vi "Multiple Files Handler.vi"(8 "Error In":errorcluster, 11 "TDMS Log":refnum<class "TDMS Logger.lvclass">) -> (0 "Error Out":errorcluster, 3 "TDMS Log Out":refnum<class "TDMS Logger.lvclass">)   [LabVIEW 2019, in "TDMS Logger.lvlib" / "TDMS Logger.lvclass"]
uses:
  TDMS Logger.lvclass
  TDMS Logger.lvclass/TDMS Logger.ctl
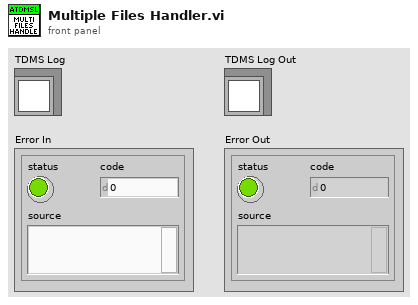
[diagram p1: front panel]
types:
  T1 = typedef "TDMS Logger.lvlib/TDMS Logger.lvclass/Multiple Files Action.ctl" = enum16{"Seperate based on size", "Seperate based on time", "Single file"}
  T2 = enum16{"open", "open or create", "create or replace", "create", "open (read-only)"}
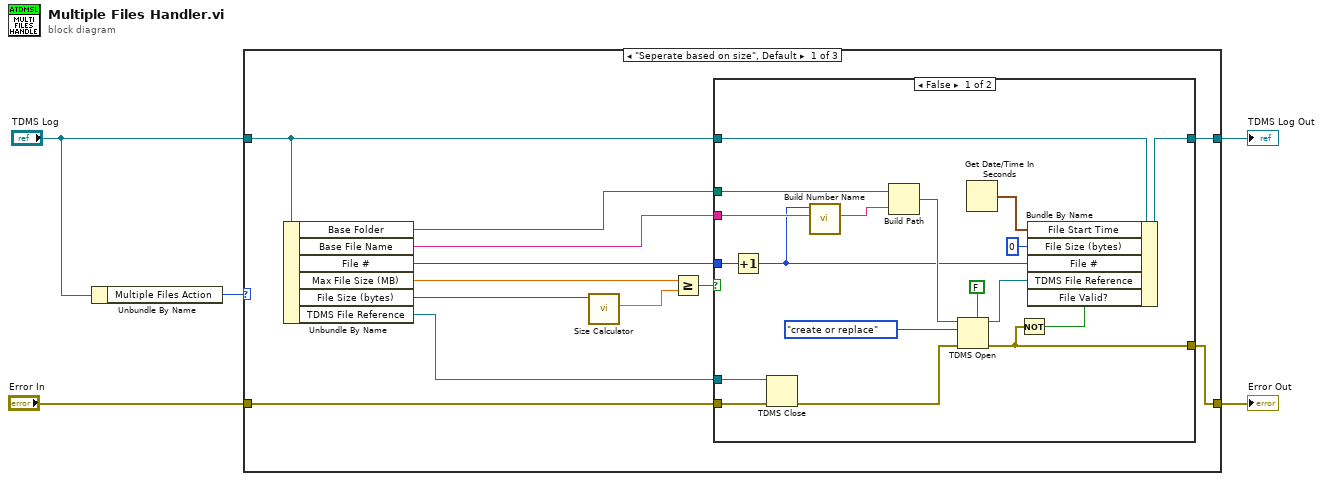
[diagram p0: block diagram]
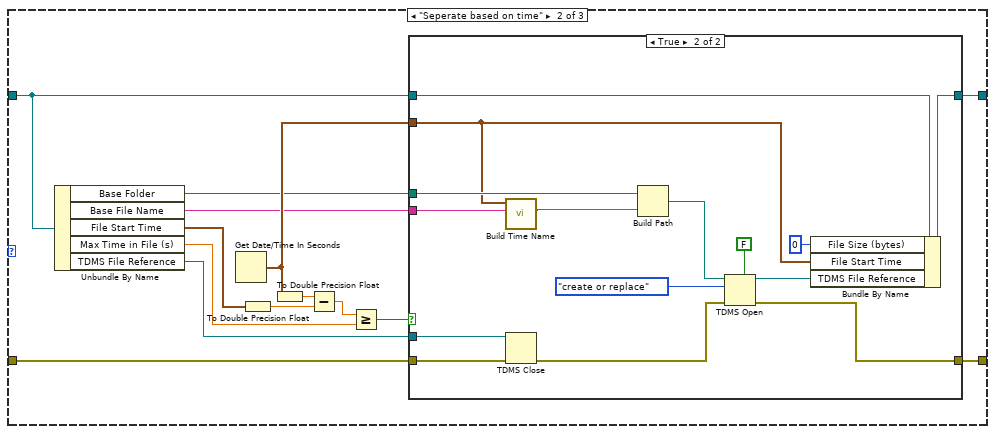
[diagram p3: hidden frame]
diagram:
  n1 = Unbundle By Name("TDMS Log") -> ("Multiple Files Action"=w5:T1)
  n2 = case shown="\"Seperate based on size\", Default" w5 {
    tunnel: [w13 w47 w70] -> w4
    tunnel: "TDMS Log" -> [w14 w48 w70]
    tunnel: "Error In" -> [w6 w46 w69]
    tunnel: [w8 w45 w69] -> w1
    frame "Seperate based on size", Default {
      n3 = Unbundle By Name(w14) -> ("Base Folder"=w9:path, "Base File Name"=w10:string, "File #"=w12:u32, "Max File Size (MB)"=w17:dbl, "File Size (bytes)"=w7:u64, "TDMS File Reference"=w11:refnum<k34>)
      n4 = call "Size Calculator.vi"("Bytes"=w7) -> ("Megabytes"=w16:dbl)  [unwired: 8 in, 2 out]
      n5 = Greater Or Equal?(x=w17, y=w16) -> (x >= y?=w15:bool)
      n6 = case shown="False" w15 {
        tunnel: w14 -> [w35 w37]
        tunnel: [w34 w37] -> w13
        tunnel: w12 -> [w33 _]
        tunnel: w11 -> [w32 _]
        tunnel: w6 -> [w31 w36]
        tunnel: w10 -> [w24 _]
        tunnel: w9 -> [w28 _]
        tunnel: [w19 w36] -> w8
        frame False {
          n7 = Increment(x=w33) -> (x+1=w22:u32)
          n8 = TDMS Close(8:w31, 11:w32) -> (0:w30:errorcluster)  [unwired: 1 out]
          n9 = call "Build Number Name.vi"("Base File Name"=w24, "File #"=w22) -> ("Numbered Name"=w23:string)  [unwired: 9 in]
          n10 = Build Path(base path=w28, name or relative path=w23) -> (appended path=w26:path)
          n11 = TDMS Open(5:FALSE ("create index file? (T)"), 8:w30, 10:T2."create or replace" ("operation (0:open)"), 11:w26) -> (0:w19:errorcluster, 3:w27:refnum<k34>)  [unwired: 3 in]
          n12 = Get Date/Time In Seconds() -> (seconds since 1Jan1904=w20:timestamp)
          n13 = Not(x=w19) -> (.not. x?=w18:bool)
          n14 = Bundle By Name(cluster=w35, "File Start Time"=w20, "File Size (bytes)"=u64 0, "File #"=w22, "TDMS File Reference"=w27, "File Valid?"=w18) -> (w34:refnum<class "TDMS Logger.lvclass">)
        }
        frame True {
        }
      }
    }
    frame "Seperate based on time" {
      n15 = Unbundle By Name(w48) -> ("Base Folder"=w41:path, "Base File Name"=w40:string, "File Start Time"=w51:timestamp, "Max Time in File (s)"=w50:dbl, "TDMS File Reference"=w44:refnum<k34>)
      n16 = Get Date/Time In Seconds() -> (seconds since 1Jan1904=w42:timestamp)
      n17 = To Double Precision Float(number=w51) -> (double precision float=w39:dbl)
      n18 = To Double Precision Float(number=w42) -> (double precision float=w38:dbl)
      n19 = Subtract(x=w38, y=w39) -> (x-y=w49:dbl)
      n20 = Greater Or Equal?(x=w49, y=w50) -> (x >= y?=w43:bool)
      n21 = case shown="True" w43 {
        tunnel: w48 -> [w53 w68]
        tunnel: [w53 w67] -> w47
        tunnel: w44 -> [_ w66]
        tunnel: w46 -> [w52 w65]
        tunnel: [w52 w60] -> w45
        tunnel: w42 -> [_ w55]
        tunnel: w41 -> [_ w58]
        tunnel: w40 -> [_ w57]
        frame False {
        }
        frame True {
          n22 = call "Build Time Name.vi"("Base File Name"=w57, "Timestamp"=w55) -> ("Time Name"=w56:string)  [unwired: 9 in]
          n23 = TDMS Close(8:w65, 11:w66) -> (0:w64:errorcluster)  [unwired: 1 out]
          n24 = Build Path(base path=w58, name or relative path=w56) -> (appended path=w61:path)
          n25 = TDMS Open(5:FALSE ("create index file? (T)"), 8:w64, 10:T2."create or replace" ("operation (0:open)"), 11:w61) -> (0:w60:errorcluster, 3:w62:refnum<k34>)  [unwired: 3 in]
          n26 = Bundle By Name(cluster=w68, "File Size (bytes)"=u64 0, "File Start Time"=w55, "TDMS File Reference"=w62) -> (w67:refnum<class "TDMS Logger.lvclass">)
        }
      }
    }
    frame "Single file" {
    }
  }
  "TDMS Log Out" <- w4
  "Error Out" <- w1
